vi "clear Session Data.vi"(0 "Session in":refnum<class "Execution.lvclass">, 11 "error in":errorcluster) -> (4 "Session out":refnum<class "Execution.lvclass">, 15 "error out":errorcluster)   [LabVIEW 2019, in "HTS.lvlib" / "Execution.lvclass"]
uses:
  Execution.lvclass
  SequenceFile/SequenceFile.lvclass
  SequenceFile/Typedefs/Session Handle.ctl
  VariableContainer/VariableContainer.lvclass
  VariableContainer/Typedefs/Session Handle.ctl
  Program Files (x86)/National Instruments/LabVIEW 2020/user.lib/_Session Fwk/Session - Root.lvclass
  cdad65d3-07d4-44e1-92f4-99dc895b8774.vi
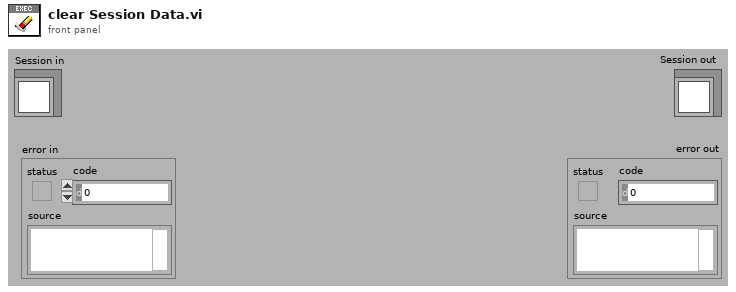
[diagram p1: front panel]
types:
  T1 = typedef "HTS.lvlib/VariableContainer.lvclass/Session Handle.ctl" = refnum<data-value>
  T2 = typedef "HTS.lvlib/SequenceFile.lvclass/Session Handle.ctl" = refnum<data-value>
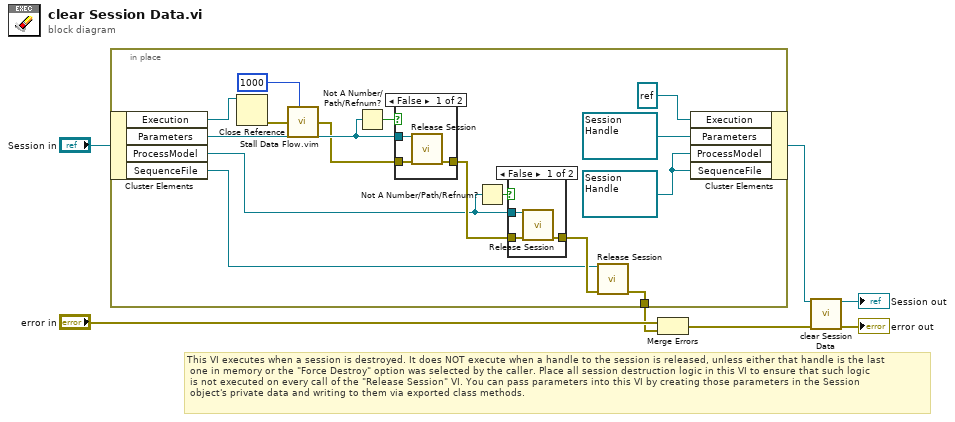
[diagram p0: block diagram]
diagram:
  # "This VI executes when a session is destroyed. It does NOT execute when a handle to the session is released, unless either that handle is the last\n one in memory or the \"Force Destroy\" option was selected by the caller. Place all session destruction logic in this VI to ensure that such logic\n is not executed on every call of the \"Release Session\" VI. You can pass parameters into this VI by creating those parameters in the Session \n object's private data and writing to them via exported class methods."
  n1 = in-place {
    in-place-border: [w11] -> w1
    w14 = T2 refnum ("SequenceFile")
    n2 = in-place-cluster #1("Session in") -> ("Execution"=w17:refnum<k7>, "Parameters"=w18:T1, "ProcessModel"=w16:T2, "SequenceFile"=w15:T2)
    n3 = Close Reference(reference=w17) -> (error out=w10:errorcluster)  [unwired: 1 in]
    n4 = call "Stall Data Flow.vim"("value in"=w10, "milliseconds to wait"=u32 1000) -> ("value out"=w9:errorcluster)  [unwired: 1 out]
    n5 = Not A Number/Path/Refnum?(number/path/refnum=w18) -> (NaN/Path/Refnum?=w20:bool)
    n6 = case shown="False" w20 {
      tunnel: w9 -> [w29 w30]
      tunnel: [w28 w30] -> w22
      tunnel: w18 -> [w27 _]
      frame False {
        n7 = call "Release Session.vi"("Session Handle"=w27, "error in (no error)"=w29) -> ("error out"=w28:errorcluster)  [unwired: 13 in]
      }
      frame True {
      }
    }
    n8 = Not A Number/Path/Refnum?(number/path/refnum=w16) -> (NaN/Path/Refnum?=w19:bool)
    n9 = case shown="False" w19 {
      tunnel: w16 -> [w25 _]
      tunnel: w22 -> [w24 w26]
      tunnel: [w23 w26] -> w21
      frame False {
        n10 = call "Release Session.vi"("Session Handle"=w25, "error in (no error)"=w24) -> ("error out"=w23:errorcluster)  [unwired: 13 in]
      }
      frame True {
      }
    }
    n11 = call "Release Session.vi"("Session Handle"=w15, "error in (no error)"=w21) -> ("error out"=w11:errorcluster)  [unwired: 13 in]
    n12 = in-place-cluster #1("Execution"=refnum<k7> refnum, "Parameters"=T1 refnum, "ProcessModel"=w14, "SequenceFile"=w14) -> (w3:refnum<class "Execution.lvclass">)
  }
  n13 = Merge Errors("error in", w1) -> (w2:errorcluster)
  n14 = call-parent "clear Session Data.vi"("OBJ - Measurement Session in"=w3, "error in"=w2) -> ("OBJ - Measurement Session out"=→"Session out":refnum<class "Execution.lvclass">, "error out"=→"error out":errorcluster)  [unwired: 12 in]
